vi "Update UI.vi"(0 "Stage Controller in":refnum<class "Stage Controller.lvclass">, 5 "Stage X Position":dbl format="%#_13g", 7 "Stage Y Position":dbl format="%#_13g", 9 "Stage Z Position":dbl format="%#_13g", 11 "error in (no error)":errorcluster) -> (4 "Stage Controller out":refnum<class "Stage Controller.lvclass">, 15 "error out":errorcluster)   [LabVIEW 2020, in "Stage.lvlib" / "Stage Controller.lvlib" / "Stage Controller.lvclass"]
uses:
  Stage Controller.lvclass
  Stage Controller.lvclass/Stage Controller.ctl
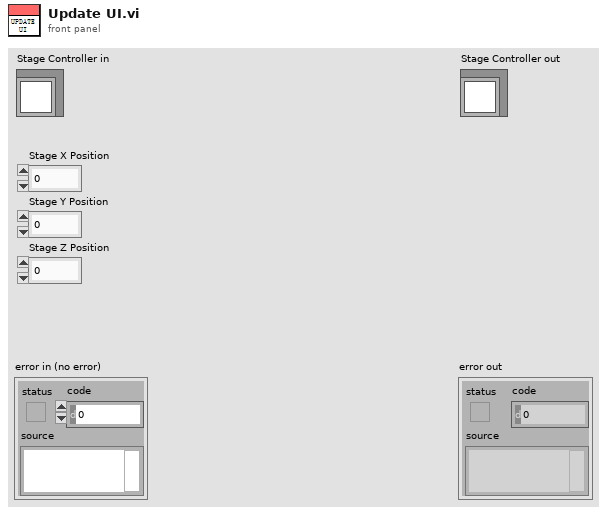
[diagram p1: front panel]
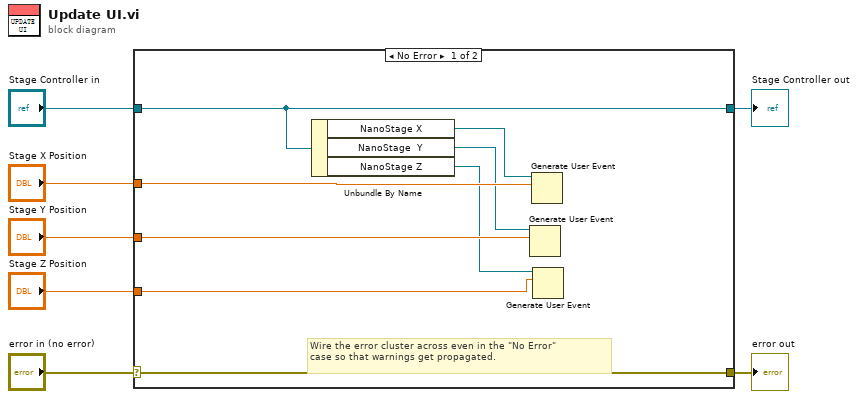
[diagram p0: block diagram]
diagram:
  n1 = case shown="No Error" "error in (no error)" {
    selector: "error in (no error)" -> [w15 w17]
    tunnel: [w15 w17] -> w6
    tunnel: [w13 w16] -> w4
    tunnel: "Stage Controller in" -> [w13 w16]
    tunnel: "Stage X Position" -> [w12 _]
    tunnel: "Stage Y Position" -> [w10 _]
    tunnel: "Stage Z Position" -> [w8 _]
    frame No Error {
      # "Wire the error cluster across even in the \"No Error\"\ncase so that warnings get propagated."
      n2 = Unbundle By Name(w13) -> ("NanoStage X"=w14:refnum<user-event>, "NanoStage  Y"=w11:refnum<user-event>, "NanoStage Z"=w9:refnum<user-event>)
      n3 = Generate User Event(user event=w11, event data cluster=w10) -> ()  [unwired: 2 in, 2 out]
      n4 = Generate User Event(user event=w14, event data cluster=w12) -> ()  [unwired: 2 in, 2 out]
      n5 = Generate User Event(user event=w9, event data cluster=w8) -> ()  [unwired: 2 in, 2 out]
    }
    frame Error {
    }
  }
  "error out" <- w6
  "Stage Controller out" <- w4
